vi "Santec OCT.vi"() -> ()   [LabVIEW 2014]
doc: "I. Description:\nThis example demonstrates how to acquire a continuous amount of data (Waveform) using the DAQ device's internal clock.\n\nII. Instructions for Running:\n1. Create an analog input voltage channel.\n2. Set the rate for the sample clock. Additionally, define the sample mode to be continuous.\n3. Call the Start VI to start the acquisition.\n4. Read the waveform data in a loop until the user hits the stop button or an error occurs.\nNote: This example reads data from one or more channels and returns an array of data. Use the Index Array function to access an individual channel of data.\n5. Call the Clear Task VI to clear the Task.\n6. Use the popup dialog box to display an error if any.\n\nIV. I/O Connections Overview:\nMake sure your signal input terminal matches the Physical Channel I/O Control. For further connection information, refer to your hardware reference manual."
uses:
  Type Defs/OCT DAQ Channel Data Type.ctl
  Type Defs/OCT Hardware States.ctl
  Classes/Galvo/Scanning Cluster.ctl
  Classes/DAQ/DAQ Parameters.ctl
  Classes/DAQ/Trigger Source.ctl
  Classes/DAQ/Trigger Slope.ctl
  Classes/DAQ/Clock Control.ctl
  Classes/Galvo/NI Galvo/NI Galvo.lvclass
  Processing Class/Intensity/Intensity Processing.lvclass
  Classes/Laser/Santec/HSL-2000/HSL-2000.lvclass
  Classes/D to A/Wavepond/Wavepond.lvclass
  Classes/DAQ/DAQ Card Options.ctl
  Classes/DAQ/ATS9462/ATS9462 Class.lvclass
  Classes/DAQ Control Functional Global States.ctl
  Classes/DAQ/ATS660/ATS660 Class.lvclass
  Classes/DAQ/DAQ Class.lvclass
  Classes/Galvo/Galvo.lvclass
panel:
  out "AFG11000 Task":refnum<k21>
  out "Alazar Task":refnum<k21>
  out "Initial DAQ Parameters":T1={"Points Per A-Scan"=1024, "A-Scans Per B-Scan"=250, "Number of B-Scans"=1, "A-Scans Per Transfer"=1, "Trigger Voltage"=0.0, "Trigger Source"=enum."External", "Trigger Slope"=enum."Rising", "Channel"=enum."Channel 1", "Clock"=enum."Internal Clock", "Bits per Sample"=0.0, "Range"=0.0}
  in  "Laser Status":string
  in  "Scanning Parameters":T6={"Fast Axis Offset"=0.0, "Slow Axis Offset"=0.0, "Slow Axis Amp"=2.0, "Fast Axis Amp"=2.0, "Scan Pattern"=enum."Raster"} {"Fast Axis Amp" max=20 format="%#.2f"; "Slow Axis Amp" max=20 format="%#.2f"; "Slow Axis Offset" max=10 format="%#.2f"; "Fast Axis Offset" max=10 format="%#.2f"}
  out "Log10?":bool
  in  "OCT Hardware States":T7
  out "Background Array":u16[](array[numeric])
  in  "Save Sweep Button":bool
  in  "Data Format":T4
  in  "Save Sweep":bool
  in  "Stop Button":bool
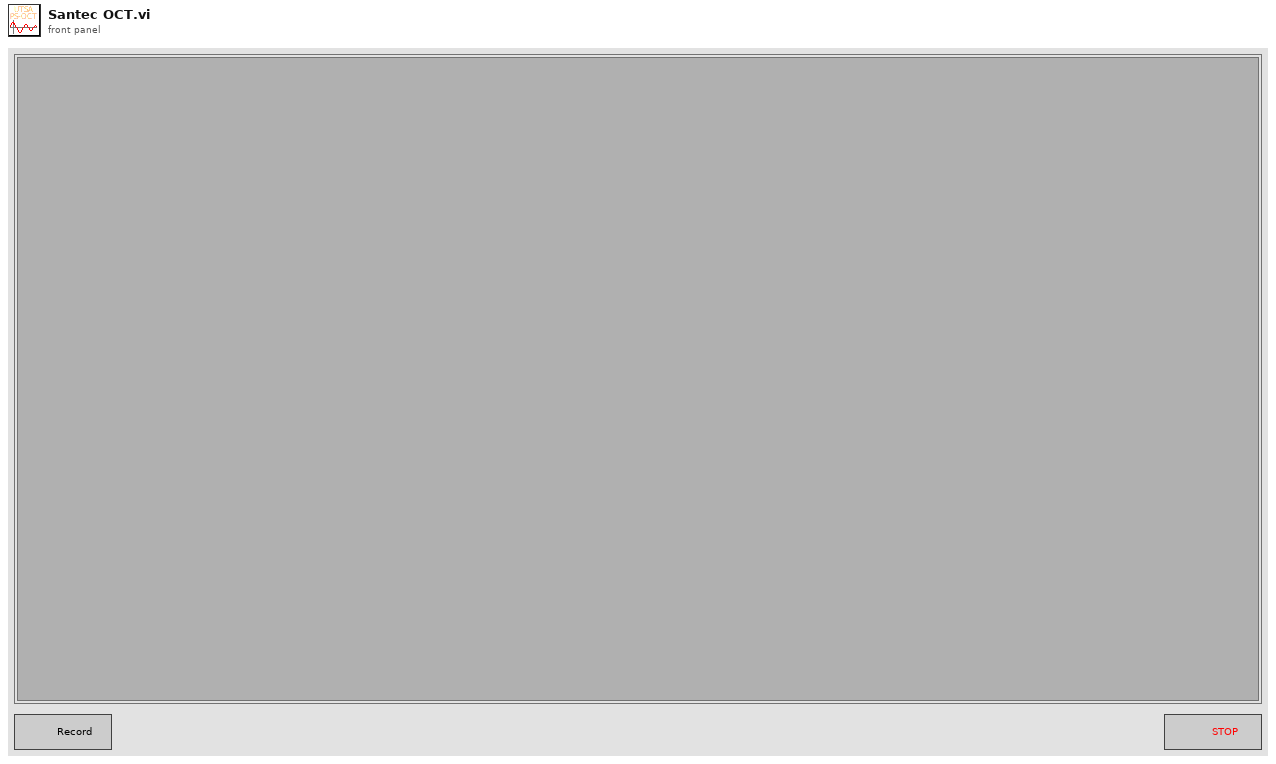
[diagram p1: front panel]
types:
  T1 = typedef "DAQ Class.lvclass/DAQ Parameters.ctl" = cluster{"Points Per A-Scan":u32, "A-Scans Per B-Scan":u32, "Number of B-Scans":u32, "A-Scans Per Transfer":u32, "Trigger Voltage":sgl, "Trigger Source":T2, "Trigger Slope":T3, "Channel":T4, "Clock":T5, "Bits per Sample":dbl, "Range":dbl}
  T2 = typedef "DAQ Class.lvclass/Trigger Source.ctl" = enum16{"External", "Channel A", "Channel B"}
  T3 = typedef "DAQ Class.lvclass/Trigger Slope.ctl" = enum16{"Rising", "Falling"}
  T4 = typedef "OCT DAQ Channel Data Type.ctl" = enum16{"Channel 1", "Channel 2", "Channel 1 and 2"}
  T5 = typedef "DAQ Class.lvclass/Clock Control.ctl" = enum16{"Internal Clock", "External Clock"}
  T6 = typedef "Galvo.lvclass/Scanning Cluster.ctl" = cluster{"Fast Axis Offset":sgl, "Slow Axis Offset":sgl, "Slow Axis Amp":sgl, "Fast Axis Amp":sgl, "Scan Pattern":enum16{"Raster"}}
  T7 = typedef "OCT Hardware States.ctl" = enum16{"Acquire Data", "Initialize Laser", "Initialize Galvos", "Startup", "Reset DAQ", "Background Subtraction", "Acquire Background", "Update DAQ Parameters", "Stop", "Set Clock", "Initialize DAQ", "Set Resampling Array", "Save Sweep", "Configure Laser", "128 x 128", "512 x 1", "512 x 512", "Review Data"}
  T8 = typedef "DAQ Class.lvclass/DAQ Card Options.ctl" = enum16{"ATS660", "ATS9462", "ATS9350"}
  T9 = typedef "DAQ Control Functional Global States.ctl" = enum16{"Status", "Set Processing Finished", "Reset", "Clear", "Set DAQ Finished"}
  T10 = enum32{"Invalid", "Standard", "Closed", "Hidden", "Minimized", "Maximized"}
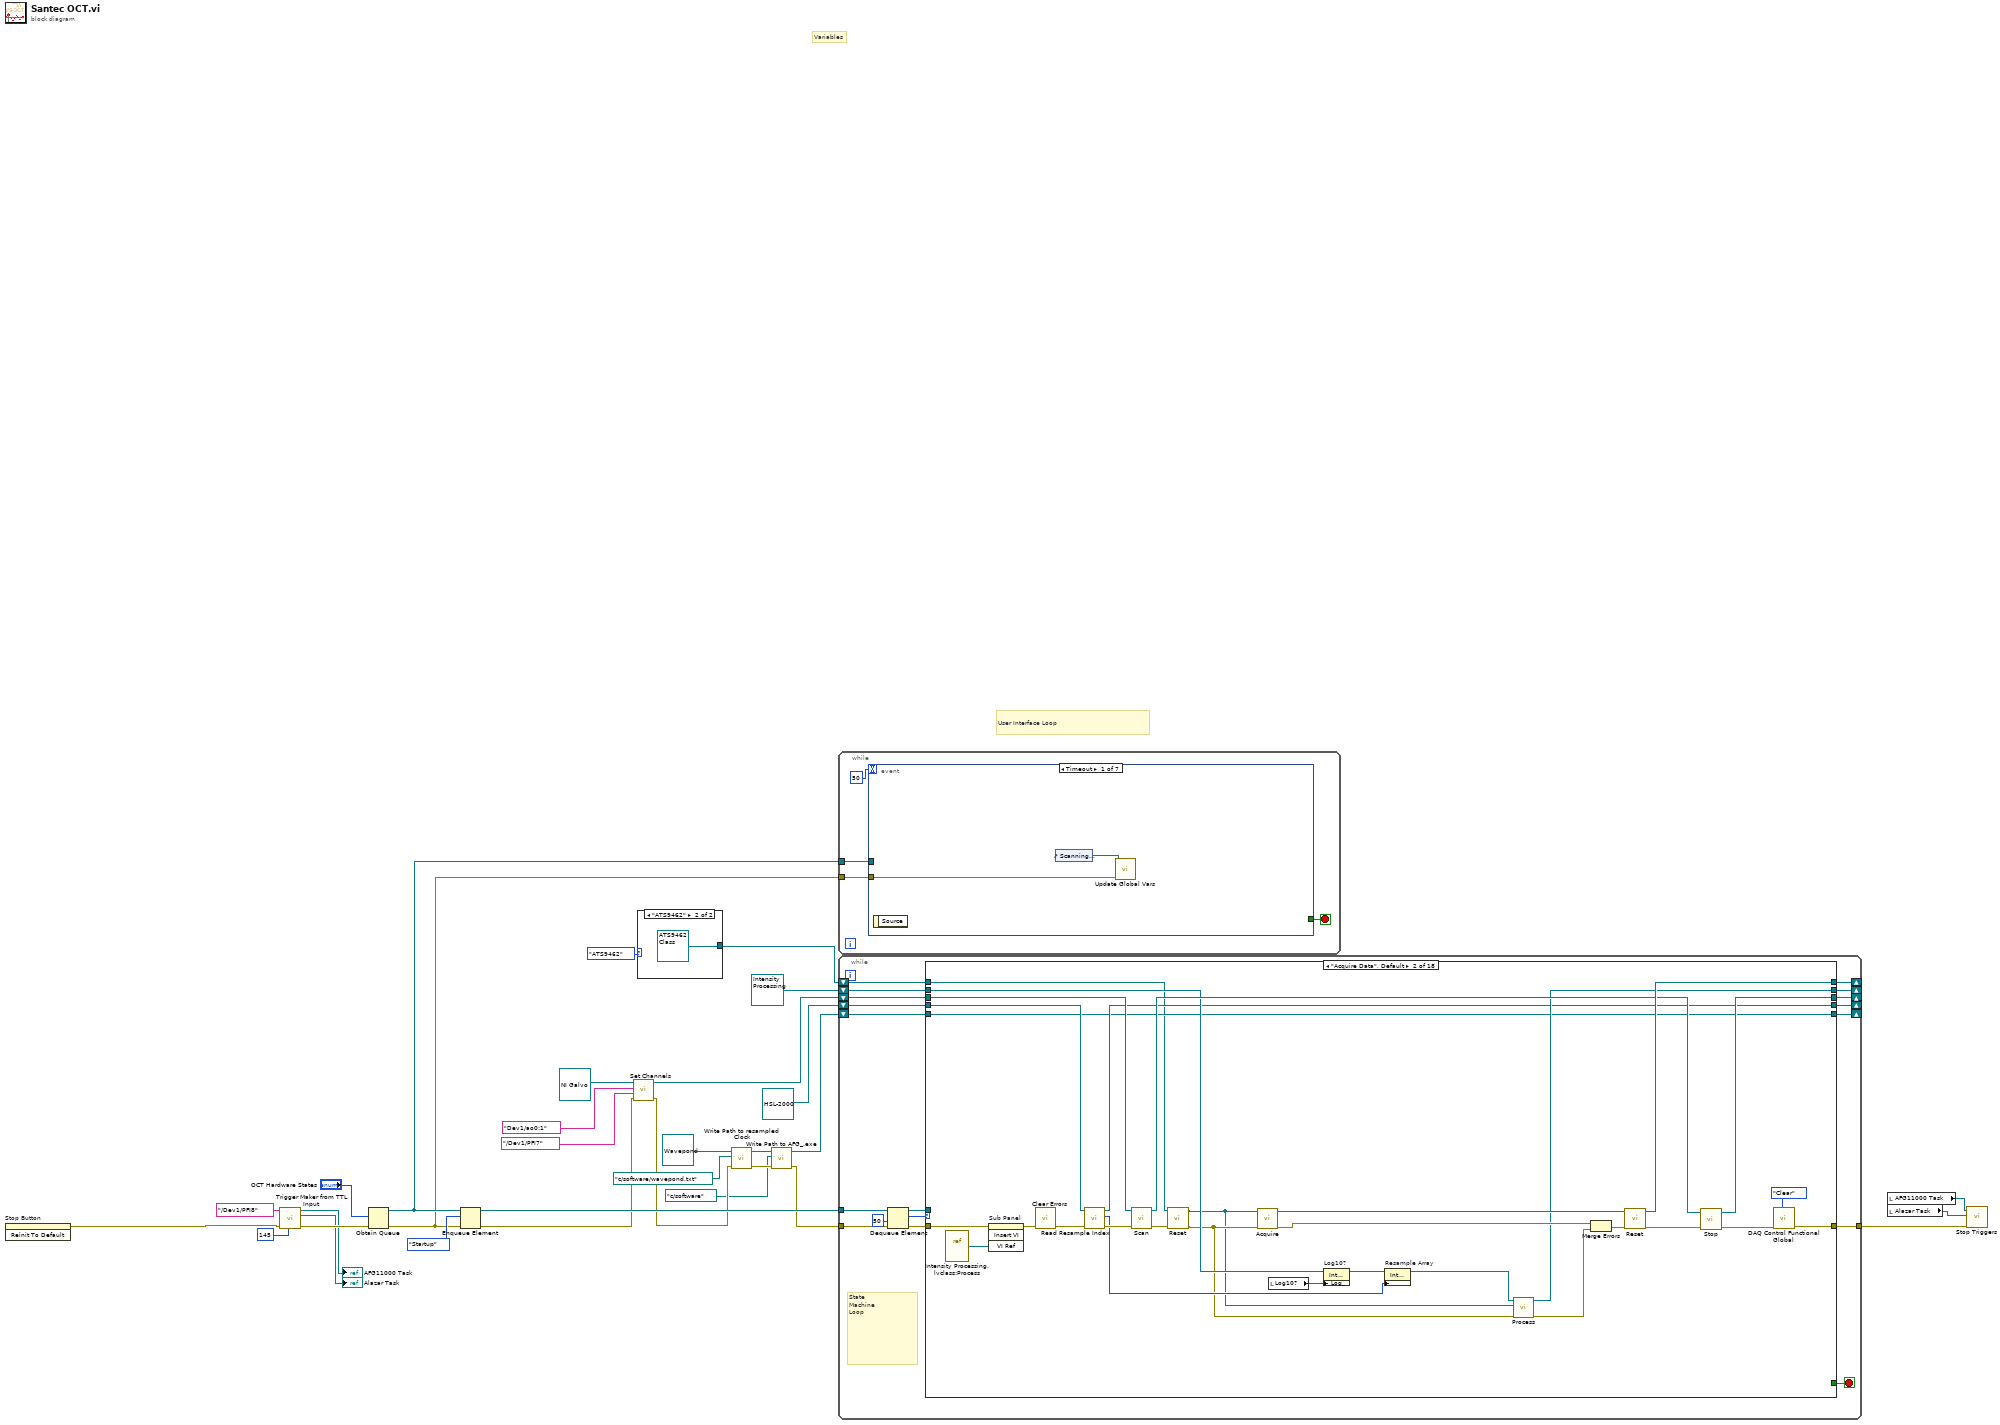
[diagram p0: block diagram]
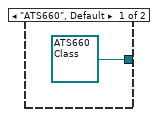
[diagram p2: hidden frame]
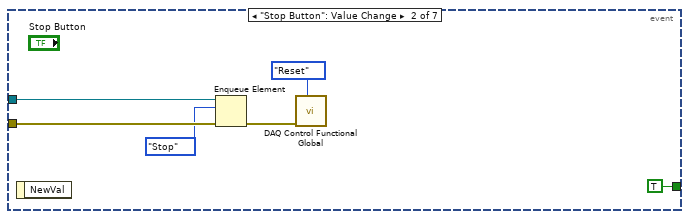
[diagram p3: hidden frame]
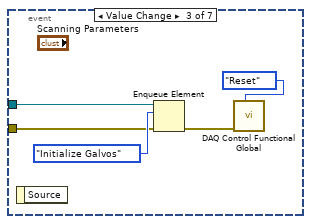
[diagram p4: hidden frame]
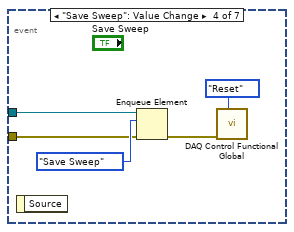
[diagram p5: hidden frame]
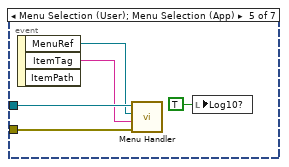
[diagram p6: hidden frame]
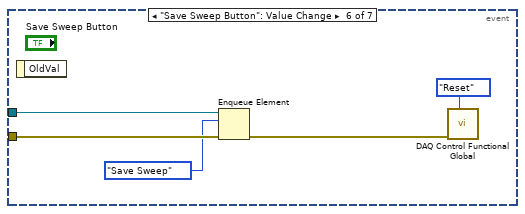
[diagram p7: hidden frame]
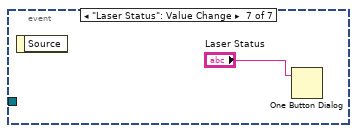
[diagram p8: hidden frame]
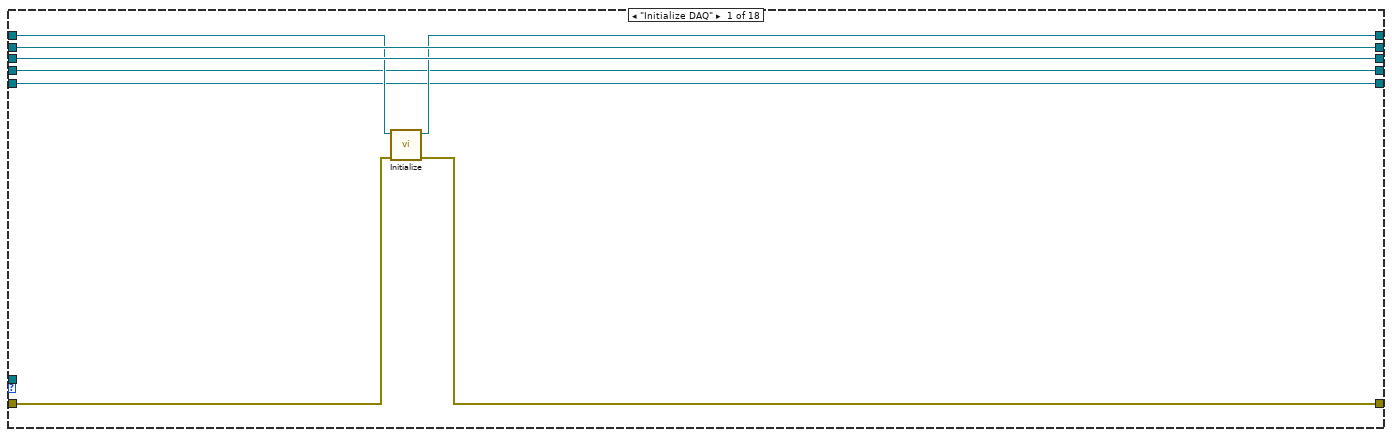
[diagram p9: hidden frame]
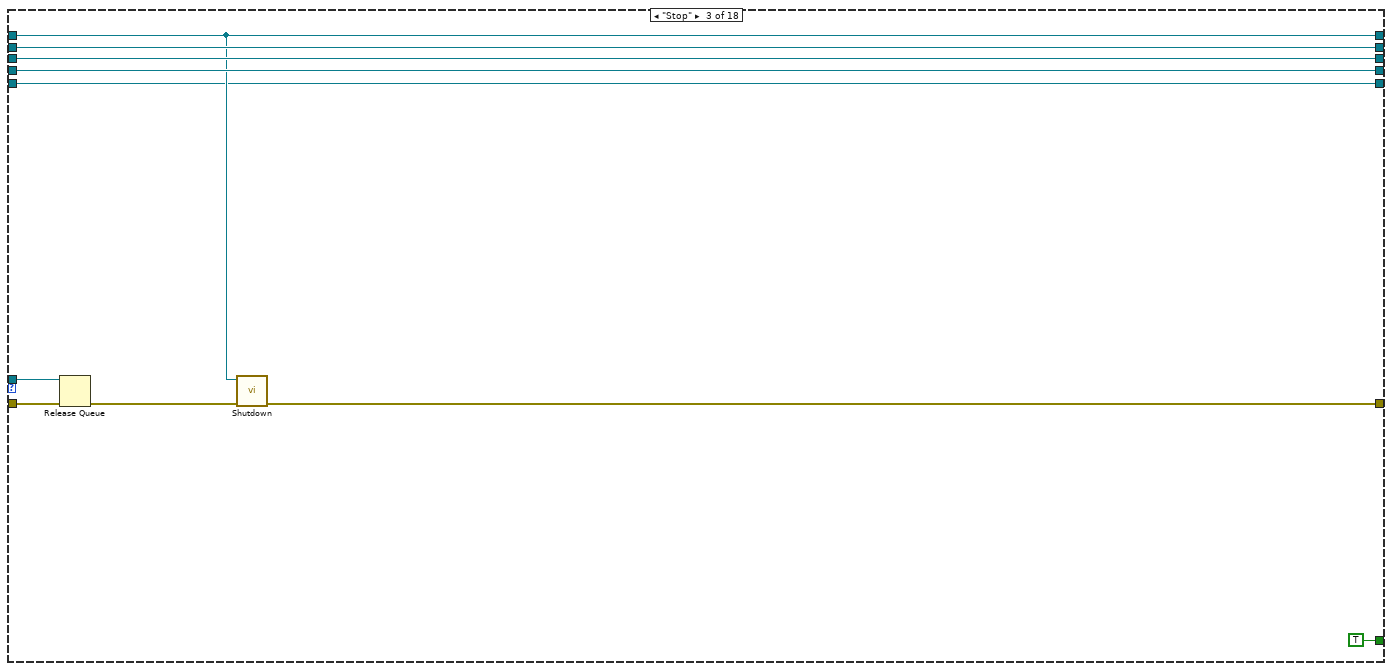
[diagram p10: hidden frame]
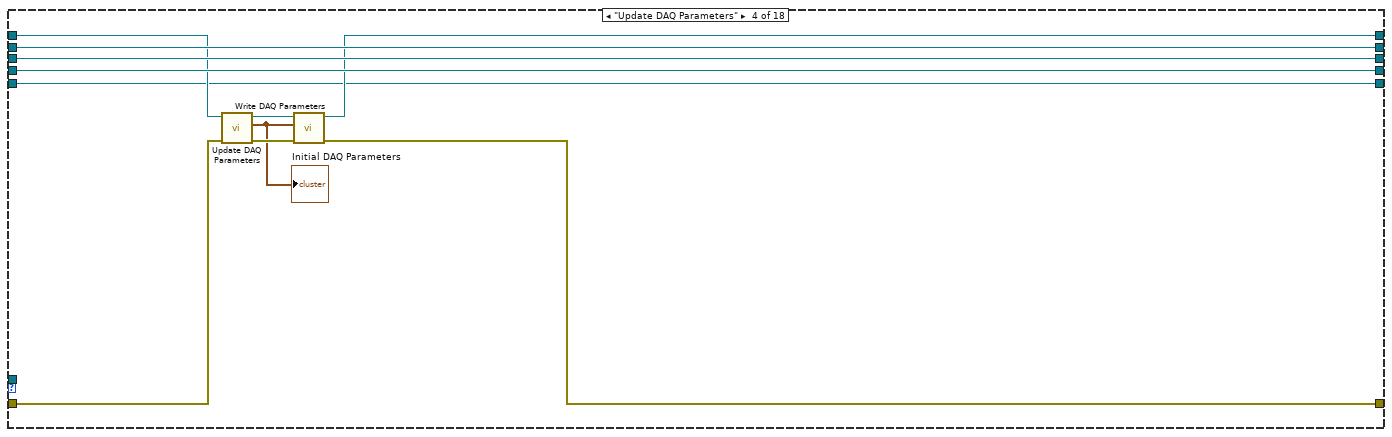
[diagram p11: hidden frame]
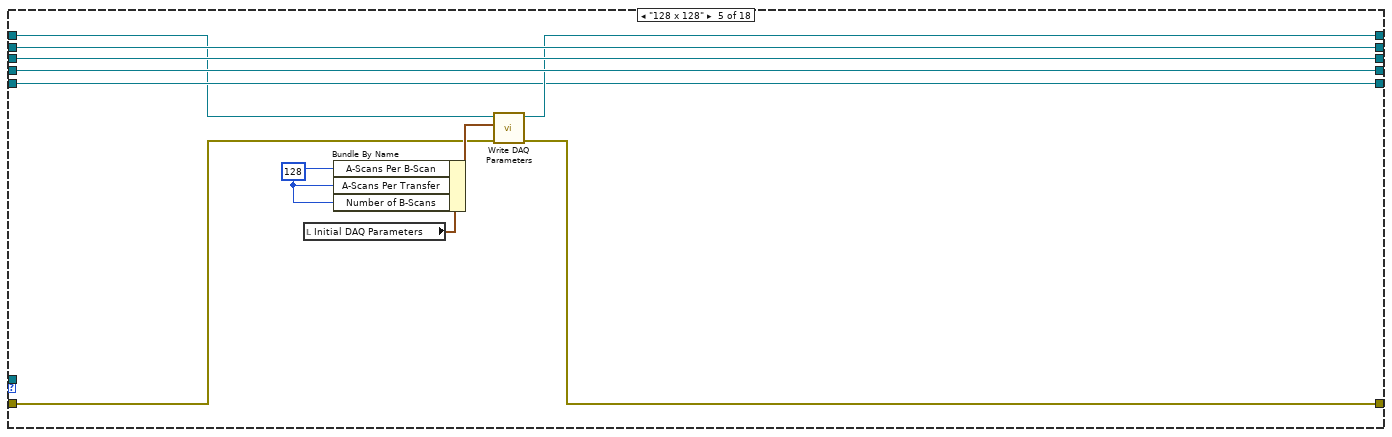
[diagram p12: hidden frame]
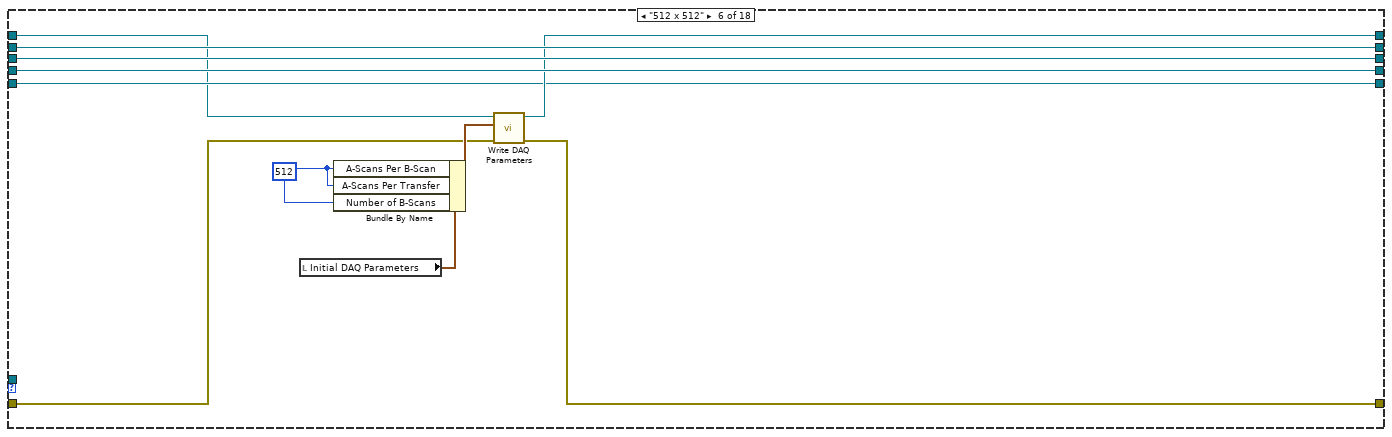
[diagram p13: hidden frame]
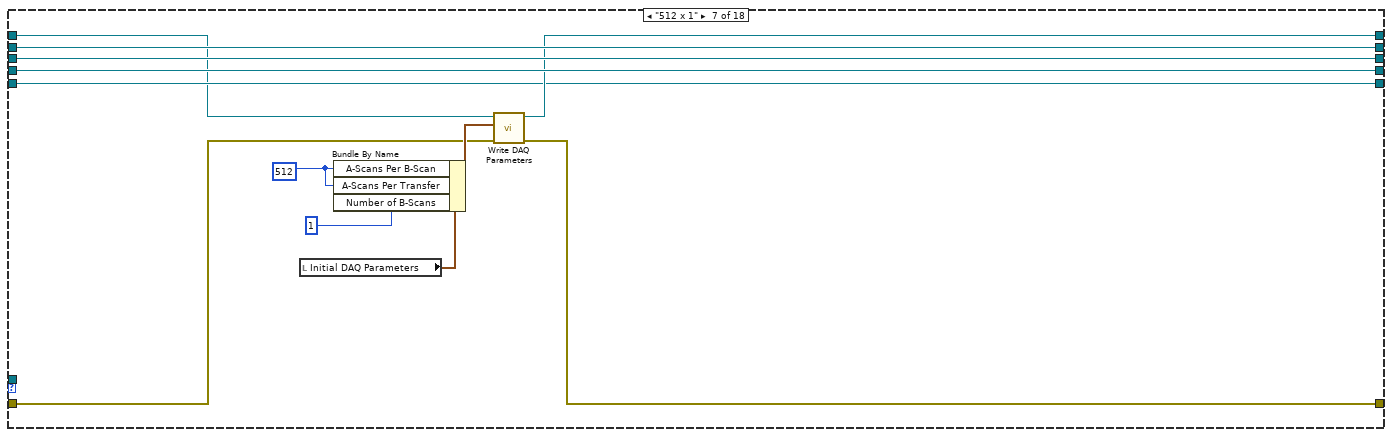
[diagram p14: hidden frame]
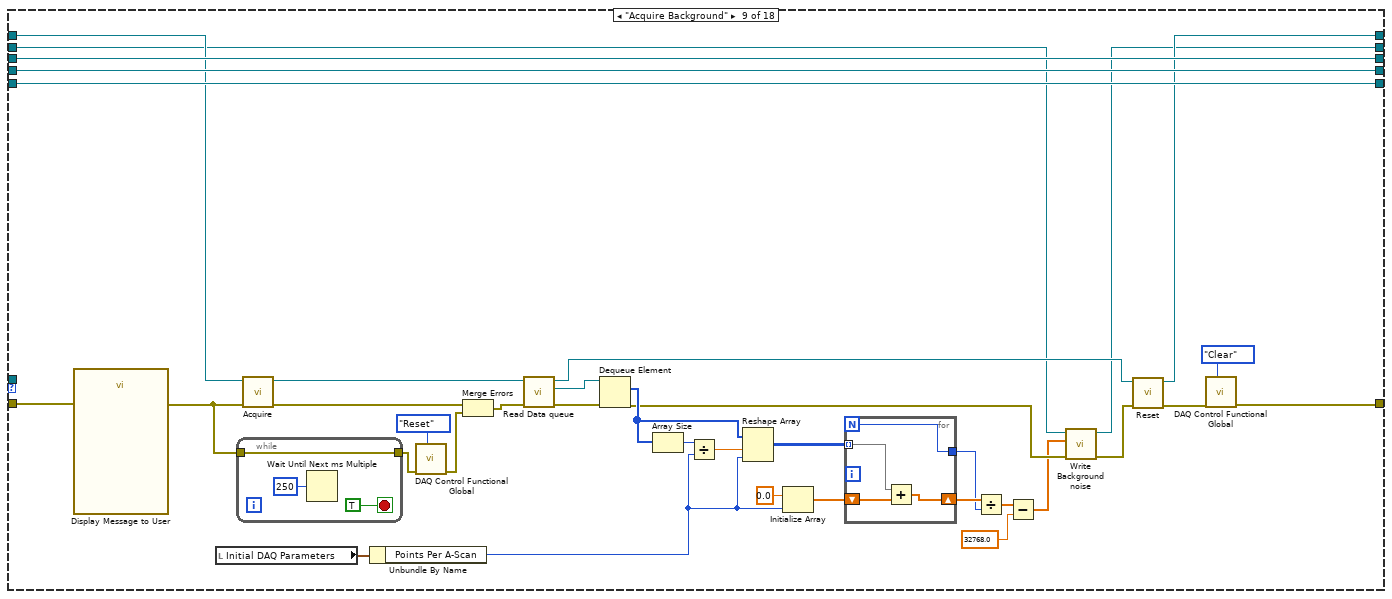
[diagram p16: hidden frame]
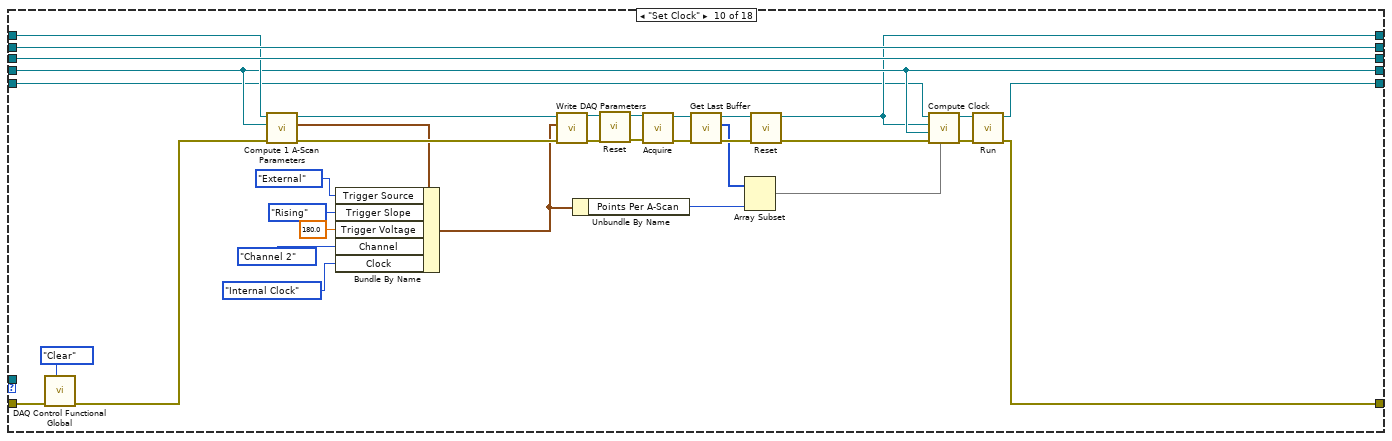
[diagram p17: hidden frame]
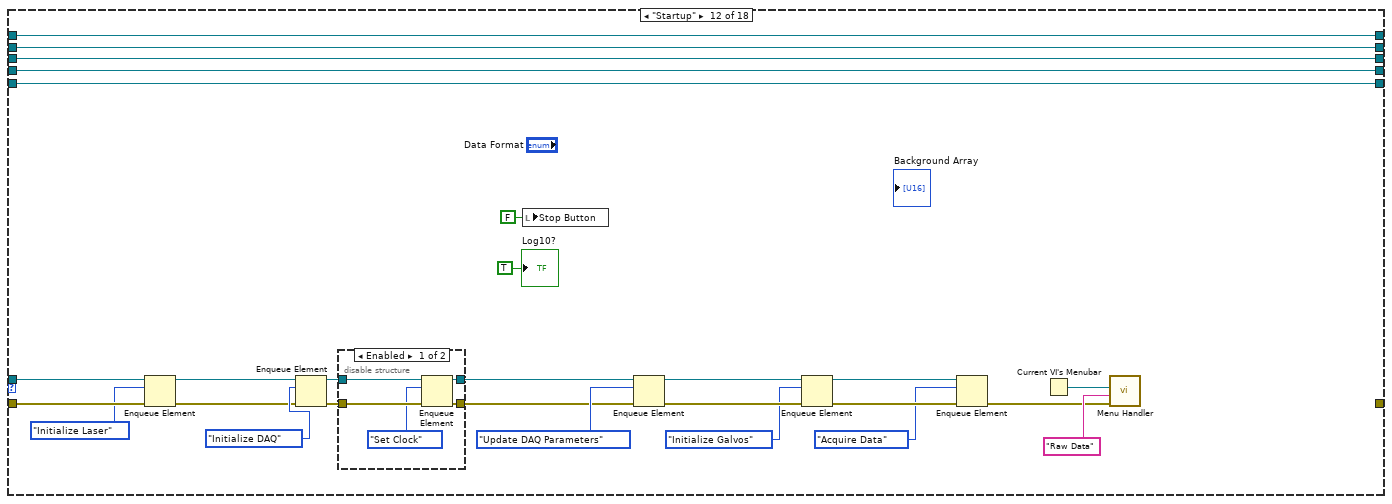
[diagram p19: hidden frame]
diagram:
  # "User Interface Loop"
  # "Variables"
  n1 = invoke on="Stop Button" class="Bool (strict)" method="Reinit To Default"() -> (error out=w1:errorcluster)  [unwired: 3 in, 2 out]
  n2 = call "Trigger Maker from TTL Input.vi"("Trigger Delay Alazar"=u32 145, "Error in"=w1, "Master Trigger In from Laser (TTL)"=tag "/Dev1/PFI8") -> ("error out"=w9:errorcluster, "Alazar Task"=→"Alazar Task":refnum<k21>, "AFG11000 Task"=→"AFG11000 Task":refnum<k21>)  [unwired: 6 in]
  n3 = Obtain Queue(element data type="OCT Hardware States", error in (no error)=w9) -> (queue out=w30:refnum<queue>, error out=w28:errorcluster)  [unwired: 3 in, 1 out]
  n4 = Enqueue Element(queue=w30, element=OCT_Hardware_States."Startup", error in (no error)=w28) -> (queue out=w21:refnum<queue>, error out=w20:errorcluster)  [unwired: 1 in, 1 out]
  n5 = call-dynamic "Set Channels.vi"("error in (no error)"=w20, "Trigger Source"=tag "/Dev1/PFI7", "Analog Output"=tag "Dev1/ao0:1", "NI Galvo in"=refnum<class "NI Galvo.lvclass"> refnum ("NI Galvo.lvclass")) -> ("error out"=w17:errorcluster, "NI Galvo out"=w25:refnum<class "NI Galvo.lvclass">)  [unwired: 6 in]
  n6 = case shown="\"ATS9462\"" DAQ_Card_Options."ATS9462" {
    tunnel: [refnum<class "ATS660 Class.lvclass"> refnum ("ATS660 Class.lvclass") refnum<class "ATS9462 Class.lvclass"> refnum ("ATS9462 Class.lvclass")] -> w22
    frame "ATS660", Default {
    }
    frame "ATS9462" {
    }
  }
  n7 = call-dynamic "Write Path to resampled Clock.vi"("error in (no error)"=w17, "Path to resampled Clock"=path "c:/software/wavepond.txt", "Wavepond in"=refnum<class "Wavepond.lvclass"> refnum ("Wavepond.lvclass")) -> ("error out"=w14:errorcluster, "Wavepond out"=w13:refnum<class "Wavepond.lvclass">)  [unwired: 7 in]
  n8 = call-dynamic "Write Path to AFG_.exe.vi"("error in (no error)"=w14, "Path to AFG*.exe"=path "c:/software" ("Path to resampled Clock"), "Wavepond in"=w13) -> ("error out"=w10:errorcluster, "Wavepond out"=w12:refnum<class "Wavepond.lvclass">)  [unwired: 7 in]
  n9 = while {
    tunnel: w21 -> [w51]
    tunnel: w10 -> [w46]
    tunnel: [w47] -> w6
    shift-right: [w43] -> _
    shift-left: w22 -> [w44]
    shift-right: [w39] -> _
    shift-left: refnum<class "Intensity Processing.lvclass"> refnum ("Intensity Processing.lvclass") -> [w42]
    shift-right: [w38] -> _
    shift-left: w25 -> [w41]
    shift-right: [w37] -> _
    shift-left: refnum<class "HSL-2000.lvclass"> refnum ("HSL-2000.lvclass") -> [w40]
    shift-right: [w34] -> _
    shift-left: w12 -> [w35]
    stop <- w36 stop-if-true
    # "State\nMachine\nLoop"
    n10 = Dequeue Element(queue=w51, timeout in ms (-1)=50, error in (no error)=w46) -> (queue out=w49:refnum<queue>, element=w45:T7, error out=w50:errorcluster)  [unwired: 1 out]
    n11 = case shown="\"Acquire Data\", Default" w45 {
      tunnel: w50 -> [w54 w80 w98 w110 w112 w124 w136 _ w182 w223 _ w239 w277 w286 _ w302 w313 w321]
      tunnel: w49 -> [_ _ w99 _ _ _ _ _ _ _ _ w240 w276 _ _ _ _ _]
      tunnel: [w59 w88 w90 w101 w117 w128 w140 _ w170 w202 _ _ w275 w289 _ w300 w308 w323] -> w47
      tunnel: w44 -> [w56 w60 w93 w103 w113 w125 w137 w149 w173 w219 w231 w244 w274 w281 w297 w305 w316 w329]
      tunnel: [w55 w77 w93 w102 w118 w129 w141 w149 w172 w199 w231 w244 w273 w280 w297 w305 w316 w329] -> w43
      tunnel: w42 -> [w58 w74 w96 w106 w121 w132 w144 w148 w156 w221 w230 w243 w272 w285 w296 w304 w315 w328]
      tunnel: w41 -> [w57 w78 w95 w105 w120 w131 w143 w147 w185 w220 w229 w242 w271 w283 w295 w303 w314 w327]
      tunnel: w40 -> [w53 w69 w94 w104 w119 w130 w142 w146 w184 w200 w228 w241 w268 w284 w294 w301 w310 w326]
      tunnel: [w58 w73 w96 w106 w121 w132 w144 w148 w155 w221 w230 w243 w272 w285 w296 w304 w315 w328] -> w39
      tunnel: [w57 w75 w95 w105 w120 w131 w143 w147 w185 w220 w229 w242 w271 w282 w295 w303 w314 w327] -> w38
      tunnel: [w53 w68 w94 w104 w119 w130 w142 w146 w184 w200 w228 w241 w267 w284 w294 w299 w309 w326] -> w37
      tunnel: [_ _ TRUE _ _ _ _ _ _ _ _ _ _ _ _ _ _ _] -> w36
      tunnel: w35 -> [w52 w64 w91 w100 w116 w127 w139 w145 w183 w195 w227 w235 w265 w279 w293 w298 w306 w325]
      tunnel: [w52 w64 w91 w100 w116 w127 w139 w145 w183 w201 w227 w235 w265 w279 w293 w298 w306 w325] -> w34
      frame "Initialize DAQ" {
        n12 = call-dynamic "Initialize.vi"("error in (no error)"=w54, "DAQ Class in"=w56) -> ("error out"=w59:errorcluster, "DAQ Class out"=w55:refnum<class "DAQ Class.lvclass">)  [unwired: 8 in]
      }
      frame "Acquire Data", Default {
        n13 = vi-ref "Intensity Processing.lvclass:Process.vi"() -> (w79:refnum<vi>)
        n14 = invoke on="Sub Panel" class="SubPanel" method="Insert VI"(error in=w80, "VI Ref"=w79) -> (error out=w72:errorcluster)  [unwired: 2 in, 3 out]
        n15 = call <vilib>:"Clear Errors.vi"("error in (no error)"=w72) -> ("error out"=w71:errorcluster)  [unwired: 5 in, 1 out]
        n16 = call-dynamic "Read Resample Index.vi"("error in (no error)"=w71, "Laser in"=w69) -> ("error out"=w70:errorcluster, "Resample Index"=w66:u32[], "Laser out"=w68:refnum<class "HSL-2000.lvclass">)  [unwired: 7 in]
        n17 = call-dynamic "Scan.vi"("error in (no error)"=w70, "NI Galvo in"=w78) -> ("error out"=w63:errorcluster, "NI Galvo out"=w76:refnum<class "NI Galvo.lvclass">)  [unwired: 8 in]
        n18 = call-dynamic "Reset.vi"("error in (no error)"=w63, "DAQ Class in"=w60) -> ("error out"=w62:errorcluster, "DAQ Class out"=w61:refnum<class "DAQ Class.lvclass">)  [unwired: 8 in]
        n19 = call-dynamic "Acquire.vi"("error in (no error)"=w62, "DAQ Class in"=w61) -> ("error out"=w86:errorcluster, "DAQ Class out"=w84:refnum<class "DAQ Class.lvclass">)  [unwired: 8 in]
        n20 = local read "Log10?"() -> (w83:bool)
        n21 = property on="Log10?" class="Intensity Processing.lvclass"(reference=w74, "Log_"=w83) -> (reference out=w67:refnum<class "Intensity Processing.lvclass">)  [unwired: 1 in, 1 out]
        n22 = property on="Resample Array" class="Intensity Processing.lvclass"(reference=w67, "Resample Array"=w66) -> (reference out=w65:refnum<class "Intensity Processing.lvclass">)  [unwired: 1 in, 1 out]
        n23 = call-dynamic "Process.vi"("error in (no error)"=w62, "DAQ Class.lvclass"=w61, "Intensity Processing in"=w65) -> ("error out"=w87:errorcluster, "Intensity Processing out"=w73:refnum<class "Intensity Processing.lvclass">)  [unwired: 7 in]
        n24 = Merge Errors(w86, w87) -> (w85:errorcluster)
        n25 = call-dynamic "Reset.vi"("error in (no error)"=w85, "DAQ Class in"=w84) -> ("error out"=w82:errorcluster, "DAQ Class out"=w77:refnum<class "DAQ Class.lvclass">)  [unwired: 8 in]
        n26 = call-dynamic "Stop.vi"("error in (no error)"=w82, "NI Galvo in"=w76) -> ("error out"=w81:errorcluster, "NI Galvo out"=w75:refnum<class "NI Galvo.lvclass">)  [unwired: 8 in]
        n27 = call "DAQ Control Functional Global.vi"("State"=DAQ_Control_Functional_Global_States."Clear", "Error In"=w81) -> ("Error Out"=w88:errorcluster)  [unwired: 6 in, 3 out]
      }
      frame "Stop" {
        n28 = Release Queue(queue=w99, error in (no error)=w98) -> (error out=w97:errorcluster)  [unwired: 1 in, 2 out]
        n29 = call-dynamic "Shutdown.vi"("error in (no error)"=w97, "DAQ Class in"=w93) -> ("error out"=w90:errorcluster)  [unwired: 8 in, 1 out]
      }
      frame "Update DAQ Parameters" {
        n30 = call-dynamic "Update DAQ Parameters.vi"("error in (no error)"=w110, "DAQ Class in"=w103) -> ("error out"=w108:errorcluster, "DAQ Parameters Out"=w107:T1, "DAQ Class out"=w109:refnum<class "DAQ Class.lvclass">)  [unwired: 7 in]
        "Initial DAQ Parameters" <- w107
        n31 = call-dynamic "Write DAQ Parameters.vi"("error in (no error)"=w108, "DAQ Parameters"=w107, "DAQ Class in"=w109) -> ("error out"=w101:errorcluster, "DAQ Class out"=w102:refnum<class "DAQ Class.lvclass">)  [unwired: 7 in]
      }
      frame "128 x 128" {
        w114 = u32 128 ("A-Scans Per B-Scan")
        n32 = local read "Initial DAQ Parameters"() -> (w111:T1)
        n33 = Bundle By Name(cluster=w111, "A-Scans Per B-Scan"=w114, "A-Scans Per Transfer"=w114, "Number of B-Scans"=w114) -> (w115:T1)
        n34 = call-dynamic "Write DAQ Parameters.vi"("error in (no error)"=w112, "DAQ Parameters"=w115, "DAQ Class in"=w113) -> ("error out"=w117:errorcluster, "DAQ Class out"=w118:refnum<class "DAQ Class.lvclass">)  [unwired: 7 in]
      }
      frame "512 x 512" {
        w122 = u32 512 ("A-Scans Per B-Scan")
        n35 = local read "Initial DAQ Parameters"() -> (w123:T1)
        n36 = Bundle By Name(cluster=w123, "A-Scans Per B-Scan"=w122, "A-Scans Per Transfer"=w122, "Number of B-Scans"=w122) -> (w126:T1)
        n37 = call-dynamic "Write DAQ Parameters.vi"("error in (no error)"=w124, "DAQ Parameters"=w126, "DAQ Class in"=w125) -> ("error out"=w128:errorcluster, "DAQ Class out"=w129:refnum<class "DAQ Class.lvclass">)  [unwired: 7 in]
      }
      frame "512 x 1" {
        w133 = u32 512 ("A-Scans Per B-Scan")
        n38 = local read "Initial DAQ Parameters"() -> (w135:T1)
        n39 = Bundle By Name(cluster=w135, "A-Scans Per B-Scan"=w133, "A-Scans Per Transfer"=w133, "Number of B-Scans"=u32 1) -> (w138:T1)
        n40 = call-dynamic "Write DAQ Parameters.vi"("error in (no error)"=w136, "DAQ Parameters"=w138, "DAQ Class in"=w137) -> ("error out"=w140:errorcluster, "DAQ Class out"=w141:refnum<class "DAQ Class.lvclass">)  [unwired: 7 in]
      }
      frame "Background Subtraction" {
      }
      frame "Acquire Background" {
        n41 = call "Display Message to User"("error in (no error)"=w182) -> ("error out"=w181:errorcluster)  [unwired: 9 in, 1 out]
        n42 = local read "Initial DAQ Parameters"() -> (w169:T1)
        n43 = while {
          tunnel: w181 -> [w190]
          tunnel: [w190] -> w158
          stop <- TRUE stop-if-true
          n44 = Wait Until Next ms Multiple(millisecond multiple=u32 250) -> ()  [unwired: 1 out]
        }
        n45 = call-dynamic "Acquire.vi"("error in (no error)"=w181, "DAQ Class in"=w173) -> ("error out"=w180:errorcluster, "DAQ Class out"=w179:refnum<class "DAQ Class.lvclass">)  [unwired: 8 in]
        n46 = Unbundle By Name(w169) -> ("Points Per A-Scan"=w165:u32)
        n47 = call "DAQ Control Functional Global.vi"("State"=DAQ_Control_Functional_Global_States."Reset", "Error In"=w158) -> ("Error Out"=w157:errorcluster)  [unwired: 6 in, 3 out]
        n48 = Merge Errors(w180, w157) -> (w178:errorcluster)
        n49 = call-dynamic "Read Data queue.vi"("error in (no error)"=w178, "DAQ Class in"=w179) -> ("error out"=w176:errorcluster, "Data queue"=w177:refnum<queue>, "DAQ Class out"=w171:refnum<class "DAQ Class.lvclass">)  [unwired: 7 in]
        n50 = Dequeue Element(queue=w177, error in (no error)=w176) -> (element=w167:u16[], error out=w154:errorcluster)  [unwired: 1 in, 2 out]
        n51 = Array Size(array=w167) -> (size(s)=w168:i32)
        n52 = Divide(x=w168, y=w165) -> (x/y=w166:dbl)
        n53 = Reshape Array(w167, w166, w165) -> (w163:u16[][])
        n54 = Initialize Array(0.0 ("element"), w165) -> (w162:dbl[])
        n55 = for {
          N -> [w186]
          tunnel: w163 -> [w187] mode=indexing
          shift-right: [w188] -> w161
          shift-left: w162 -> [w189]
          tunnel: [w186] -> w160
          n56 = Add(x=w187, y=w189) -> (x+y=w188:dbl[])
        }
        n57 = Divide(x=w161, y=w160) -> (x/y=w152:dbl[])
        n58 = Subtract(x=w152, y=32768.0 ("element")) -> (x-y=w151:dbl[])
        n59 = call-dynamic "Write Background noise.vi"("error in (no error)"=w154, "Background noise"=w151, "Processing in"=w156) -> ("error out"=w153:errorcluster, "Processing out"=w155:refnum<class "Intensity Processing.lvclass">)  [unwired: 7 in]
        n60 = call-dynamic "Reset.vi"("error in (no error)"=w153, "DAQ Class in"=w171) -> ("error out"=w174:errorcluster, "DAQ Class out"=w172:refnum<class "DAQ Class.lvclass">)  [unwired: 8 in]
        n61 = call "DAQ Control Functional Global.vi"("State"=DAQ_Control_Functional_Global_States."Clear", "Error In"=w174) -> ("Error Out"=w170:errorcluster)  [unwired: 6 in, 3 out]
      }
      frame "Set Clock" {
        n62 = call "DAQ Control Functional Global.vi"("State"=DAQ_Control_Functional_Global_States."Clear", "Error In"=w223) -> ("Error Out"=w194:errorcluster)  [unwired: 6 in, 3 out]
        n63 = call "Compute 1 A-Scan Parameters.vi"("error in (no error)"=w194, "Laser In"=w200, "DAQ Class.lvclass"=w219) -> ("error out"=w222:errorcluster, "DAQ Parameters"=w218:T1, "DAQ Class.lvclass 2"=w204:refnum<class "DAQ Class.lvclass">)  [unwired: 6 in]
        n64 = Bundle By Name(cluster=w218, "Trigger Source"=Trigger_Source."External", "Trigger Slope"=Trigger_Slope."Rising", "Trigger Voltage"=sgl 180.0, "Channel"=OCT_DAQ_Channel_Data_Type."Channel 2", "Clock"=Clock_Control."Internal Clock") -> (w212:T1)
        n65 = call-dynamic "Write DAQ Parameters.vi"("error in (no error)"=w222, "DAQ Parameters"=w212, "DAQ Class in"=w204) -> ("error out"=w207:errorcluster, "DAQ Class out"=w206:refnum<class "DAQ Class.lvclass">)  [unwired: 7 in]
        n66 = Unbundle By Name(w212) -> ("Points Per A-Scan"=w210:u32)
        n67 = call-dynamic "Reset.vi"("error in (no error)"=w207, "DAQ Class in"=w206) -> ("error out"=w209:errorcluster, "DAQ Class out"=w208:refnum<class "DAQ Class.lvclass">)  [unwired: 8 in]
        n68 = call-dynamic "Acquire.vi"("error in (no error)"=w209, "DAQ Class in"=w208) -> ("error out"=w225:errorcluster, "DAQ Class out"=w226:refnum<class "DAQ Class.lvclass">)  [unwired: 8 in]
        n69 = call-dynamic "Get Last Buffer.vi"("error in (no error)"=w225, "DAQ Class in"=w226) -> ("error out"=w216:errorcluster, "Last Buffer"=w211:u16[], "DAQ Class out"=w215:refnum<class "DAQ Class.lvclass">)  [unwired: 7 in]
        n70 = Array Subset(array=w211, length=w210) -> (w205:u16[])  [unwired: 1 in]
        n71 = call-dynamic "Reset.vi"("error in (no error)"=w216, "DAQ Class in"=w215) -> ("error out"=w198:errorcluster, "DAQ Class out"=w199:refnum<class "DAQ Class.lvclass">)  [unwired: 8 in]
        n72 = call-dynamic "Compute Clock.vi"("k-space signal in"=w205, "error in (no error)"=w198, "Laser.lvclass"=w200, "DAQ Class.lvclass"=w199, "Wavepond in"=w195) -> ("error out"=w193:errorcluster, "Wavepond out"=w203:refnum<class "Wavepond.lvclass">)  [unwired: 5 in]
        n73 = call-dynamic "Run.vi"("error in (no error)"=w193, "Wavepond in"=w203) -> ("error out"=w202:errorcluster, "Wavepond out"=w201:refnum<class "Wavepond.lvclass">)  [unwired: 8 in]
      }
      frame "Set Resampling Array" {
      }
      frame "Startup" {
        n74 = Enqueue Element(queue=w240, element=OCT_Hardware_States."Initialize Laser", error in (no error)=w239) -> (queue out=w237:refnum<queue>, error out=w238:errorcluster)  [unwired: 1 in, 1 out]
        n75 = Enqueue Element(queue=w237, element=OCT_Hardware_States."Initialize DAQ", error in (no error)=w238) -> (queue out=w248:refnum<queue>, error out=w247:errorcluster)  [unwired: 1 in, 1 out]
        n76 = disable-structure shown="Enabled" {
          disable-tunnel: w248 -> [w263 w264]
          disable-tunnel: w247 -> [w262 _]
          disable-tunnel: [w261 w264] -> w246
          disable-tunnel: [w260 _] -> w245
          frame Enabled {
            n77 = Enqueue Element(queue=w263, element=OCT_Hardware_States."Set Clock", error in (no error)=w262) -> (queue out=w261:refnum<queue>, error out=w260:errorcluster)  [unwired: 1 in, 1 out]
          }
          frame Disabled {
          }
        }
        n78 = local write "Stop Button"(FALSE ("Sweep Ready for saving")) -> ()
        n79 = Enqueue Element(queue=w246, element=OCT_Hardware_States."Update DAQ Parameters", error in (no error)=w245) -> (queue out=w256:refnum<queue>, error out=w255:errorcluster)  [unwired: 1 in, 1 out]
        n80 = Enqueue Element(queue=w256, element=OCT_Hardware_States."Initialize Galvos", error in (no error)=w255) -> (queue out=w251:refnum<queue>, error out=w250:errorcluster)  [unwired: 1 in, 1 out]
        n81 = Enqueue Element(queue=w251, element=OCT_Hardware_States."Acquire Data", error in (no error)=w250) -> (error out=w232:errorcluster)  [unwired: 1 in, 2 out]
        n82 = Current VI's Menubar() -> (w233:refnum<k9>)
        n83 = call "Menu Handler.vi"("error in (no error)"=w232, "ItemTag"="Raw Data", "Menu in"=w233) -> ()  [unwired: 7 in, 2 out]
        "Log10?" <- TRUE ("Log10?")
      }
      frame "Save Sweep" {
        n84 = Enqueue Element(queue=w276, element=OCT_Hardware_States."Acquire Data", error in (no error)=w277) -> (error out=w270:errorcluster)  [unwired: 1 in, 2 out]
        n85 = call-dynamic "Read Resample Index.vi"("error in (no error)"=w270, "Laser in"=w268) -> ("error out"=w269:errorcluster, "Resample Index"=w266:u32[], "Laser out"=w267:refnum<class "HSL-2000.lvclass">)  [unwired: 7 in]
        n86 = call-dynamic "Save.vi"("error in (no error)"=w269, "Resampling Array"=w266, "DAQ Class in"=w274) -> ("error out"=w275:errorcluster, "DAQ Class out"=w273:refnum<class "DAQ Class.lvclass">)  [unwired: 7 in]
      }
      frame "Initialize Galvos" {
        n87 = call-dynamic "Read DAQ Parameters.vi"("error in (no error)"=w286, "DAQ Class in"=w281) -> ("error out"=w287:errorcluster, "DAQ Parameters"=w288:T1, "DAQ Class out"=w280:refnum<class "DAQ Class.lvclass">)  [unwired: 7 in]
        n88 = local read "Scanning Parameters"() -> (w292:T6)
        n89 = call-dynamic "Configure.vi"("error in (no error)"=w287, "DAQ Parameters"=w288, "Scanning Parameters"=w292, "NI Galvo in"=w283) -> ("error out"=w291:errorcluster, "NI Galvo out"=w290:refnum<class "NI Galvo.lvclass">)  [unwired: 6 in]
        n90 = call-dynamic "Initialize.vi"("error in (no error)"=w291, "NI Galvo in"=w290) -> ("error out"=w289:errorcluster, "NI Galvo out"=w282:refnum<class "NI Galvo.lvclass">)  [unwired: 8 in]
      }
      frame "Reset DAQ" {
      }
      frame "Configure Laser" {
        n91 = call-dynamic "Configure.vi"("error in (no error)"=w302, "Santec in"=w301) -> ("error out"=w300:errorcluster, "Santec out"=w299:refnum<class "HSL-2000.lvclass">)  [unwired: 8 in]
      }
      frame "Initialize Laser" {
        n92 = call-dynamic "Init.vi"("error in (no error)"=w313, "HSL-2000 in"=w310) -> ("error out"=w311:errorcluster, "HSL-2000 out"=w312:refnum<class "HSL-2000.lvclass">)  [unwired: 8 in]
        n93 = call-dynamic "Read Status.vi"("error in (no error)"=w311, "Laser in"=w312) -> ("error out"=w308:errorcluster, "Status"=w307:string, "Laser out"=w309:refnum<class "HSL-2000.lvclass">)  [unwired: 7 in]
        n94 = local write "Laser Status"(w307) -> ()
      }
      frame "Review Data" {
        w324 = TRUE ("Auto Dispose Reference")
        n95 = vi-ref "Post-Processing VI Bin Files.vi"() -> (w322:refnum<vi>)
        n96 = invoke class="VI" method="FP.Open"(reference=w322, error in=w321, "Activate"=TRUE ("Activate?"), "State"=T10."Standard") -> (reference out=w319:refnum<vi>, error out=w320:errorcluster)  [unwired: 1 in, 3 out]
        n97 = invoke class="VI" method="Run VI"(reference=w319, error in=w320, "Wait until done"=w324, "Auto Dispose Ref"=w324) -> (error out=w323:errorcluster)  [unwired: 1 in, 4 out]
      }
    }
  }
  n98 = while {
    tunnel: w30 -> [w333]
    tunnel: w28 -> [w332]
    stop <- w330 stop-if-true
    n99 = event shown="[0] Timeout" {
      selector: _ -> [_ _ _ _ _ _ _]
      dyn-events: _ -> [_ _ _ _ _ _ _]
      timeout: 50 -> [_ _ _ _ _ _ _]
      tunnel: w333 -> [_ w340 w343 w348 w355 w358 _]
      tunnel: w332 -> [w334 w341 w344 w349 w356 w360 _]
      tunnel: [_ TRUE _ _ _ _ _] -> w330
      event Timeout {
        n100 = event-data() -> ()  [unwired: 1 in, 1 out]
        n101 = control-ref of="Scanning Parameters"() -> (w335:refnum<vi>)
        n102 = call "Update Global Vars.vi"("Error In"=w334, "Cluster in"=w335) -> ()  [unwired: 9 in, 1 out]
      }
      event "Stop Button": Value Change {
        n103 = event-data() -> ()  [unwired: 1 in, 1 out]
        n104 = Enqueue Element(queue=w340, element=OCT_Hardware_States."Stop", error in (no error)=w341) -> (error out=w338:errorcluster)  [unwired: 1 in, 2 out]
        n105 = call "DAQ Control Functional Global.vi"("State"=DAQ_Control_Functional_Global_States."Reset", "Error In"=w338) -> ()  [unwired: 6 in, 4 out]
      }
      event Value Change {
        n106 = event-data() -> ()  [unwired: 1 in, 1 out]
        n107 = Enqueue Element(queue=w343, element=OCT_Hardware_States."Initialize Galvos", error in (no error)=w344) -> (error out=w345:errorcluster)  [unwired: 1 in, 2 out]
        n108 = call "DAQ Control Functional Global.vi"("State"=DAQ_Control_Functional_Global_States."Reset", "Error In"=w345) -> ()  [unwired: 6 in, 4 out]
      }
      event "Save Sweep": Value Change {
        n109 = event-data() -> ()  [unwired: 1 in, 1 out]
        n110 = Enqueue Element(queue=w348, element=OCT_Hardware_States."Save Sweep", error in (no error)=w349) -> (error out=w347:errorcluster)  [unwired: 1 in, 2 out]
        n111 = call "DAQ Control Functional Global.vi"("State"=DAQ_Control_Functional_Global_States."Reset", "Error In"=w347) -> ()  [unwired: 6 in, 4 out]
      }
      event Menu Selection (User); Menu Selection (App) {
        n112 = event-data() -> ("MenuRef"=w354:refnum<k9>, "ItemTag"=w353:string)  [unwired: 1 in, 1 out]
        n113 = call "Menu Handler.vi"("error in (no error)"=w356, "ItemTag"=w353, "Menu in"=w354, "queue in"=w355) -> ()  [unwired: 6 in, 2 out]
        n114 = local write "Log10?"(TRUE ("Log10?")) -> ()
      }
      event "Save Sweep Button": Value Change {
        n115 = event-data() -> ()  [unwired: 1 in, 1 out]
        n116 = Enqueue Element(queue=w358, element=OCT_Hardware_States."Save Sweep", error in (no error)=w360) -> (error out=w359:errorcluster)  [unwired: 1 in, 2 out]
        n117 = call "DAQ Control Functional Global.vi"("State"=DAQ_Control_Functional_Global_States."Reset", "Error In"=w359) -> ()  [unwired: 6 in, 4 out]
      }
      event "Laser Status": Value Change {
        n118 = event-data() -> ()  [unwired: 1 in, 1 out]
        n119 = One Button Dialog(message="Laser Status") -> ()  [unwired: 1 in, 1 out]
      }
    }
  }
  n120 = local read "AFG11000 Task"() -> (w4:refnum<k21>)
  n121 = local read "Alazar Task"() -> (w5:refnum<k21>)
  n122 = call "Stop Triggers.vi"("Error in"=w6, "Alazar Task"=w5, "AFG11000 Task"=w4) -> ()  [unwired: 8 in, 1 out]
